vi "Configure Trigger (Edge Then Edge - Source).vi"(6 "Trigger Source Channel (0: Channel 1)":i32(ring) items=["Channel 1", "Channel 2", "Channel 3", "Channel 4", "D0", "D1", "D2", "D3", "D4", "D5", "D6", "D7", "D8", "D9", "D10", "D11", "D12", "D13", "D14", "D15"], 7 "Trigger Edge Slope (1: Positive)":i32(ring)=1 items=["Negative", "Positive"], 8 "error in (no error)":errorcluster, 9 "Arming Source Channel (0: Channel 1)":i32(ring) items=["Channel 1", "Channel 2", "Channel 3", "Channel 4", "D0", "D1", "D2", "D3", "D4", "D5", "D6", "D7", "D8", "D9", "D10", "D11", "D12", "D13", "D14", "D15"], 10 "Arming Edge Slope (1: Positive)":i32(ring)=1 items=["Negative", "Positive"], 11 "VISA resource name":refnum<visa-resource-name>) -> (0 "error out":errorcluster, 3 "VISA resource name out":refnum<visa-resource-name>)   [LabVIEW 2015, in "Agilent 2000 3000 X-Series.lvlib"]
doc: "Configures the sources of Delay(Edge Then Edge) trigger mode."
uses:
  Agilent 2000 3000 X-Series.lvlib
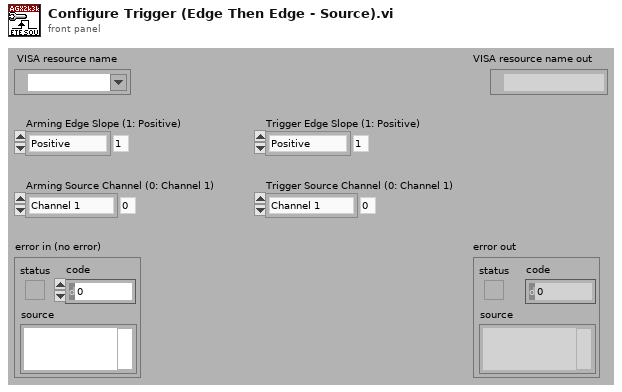
[diagram p1: front panel]
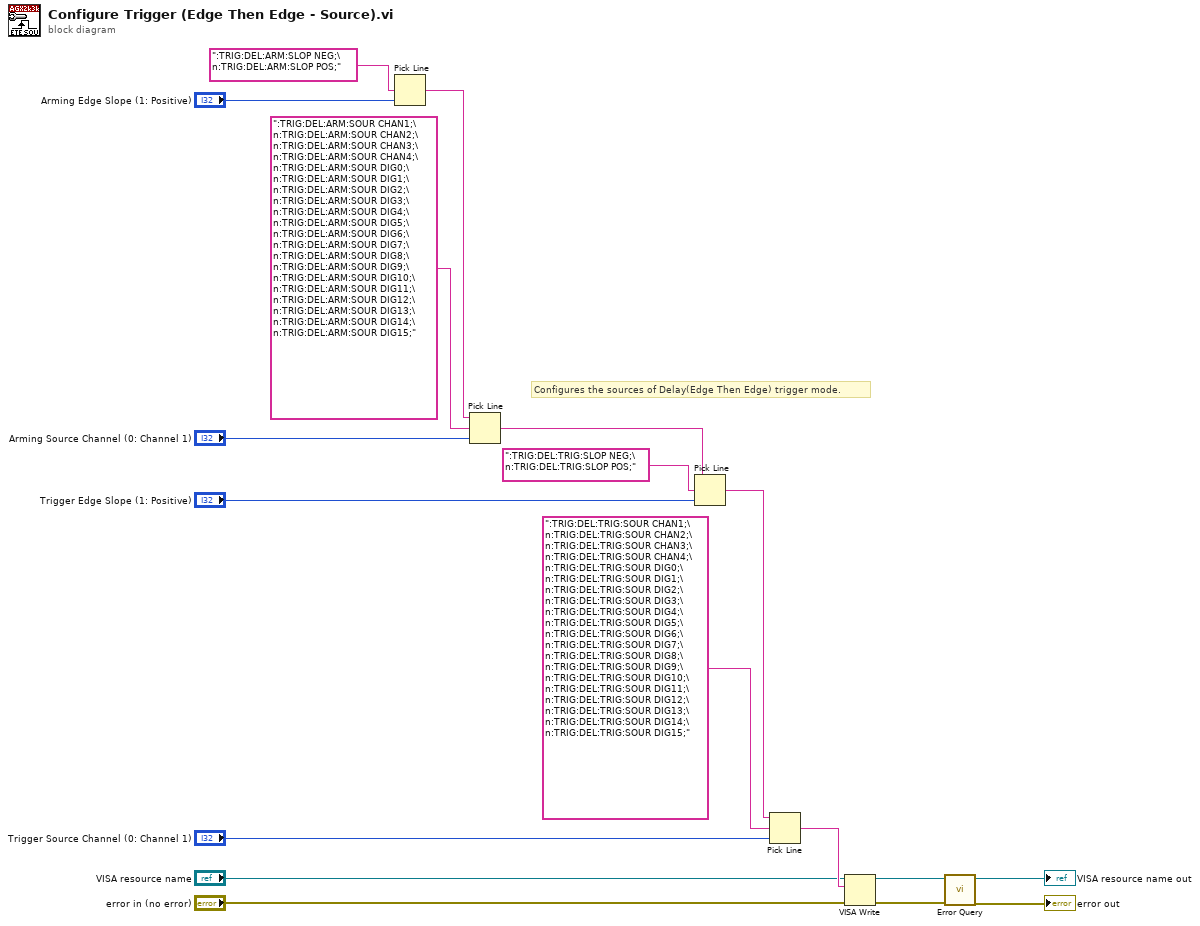
[diagram p0: block diagram]
diagram:
  # "Configures the sources of Delay(Edge Then Edge) trigger mode."
  n1 = Pick Line(multi-line string=":TRIG:DEL:ARM:SLOP NEG;\n:TRIG:DEL:ARM:SLOP POS;", line index="Arming Edge Slope (1: Positive)") -> (output string=w14:string)  [unwired: 1 out]
  n2 = Pick Line(string ("")=w14, multi-line string=":TRIG:DEL:ARM:SOUR CHAN1;\n:TRIG:DEL:ARM:SOUR CHAN2;\n:TRIG:DEL:ARM:SOUR CHAN3;\n:TRIG:DEL:ARM:SOUR CHAN4;\n:TRIG:DEL:ARM:SOUR DIG0;\n:TRIG:DEL:ARM:SOUR DIG1;\n:TRIG:DEL:ARM:SOUR DIG2;\n:TRIG:DEL:ARM:SOUR DIG3;\n:TRIG:DEL:ARM:SOUR DIG4;\n:TRIG:DEL:ARM:SOUR DIG5;\n:TRIG:DEL:ARM:SOUR DIG6;\n:TRIG:DEL:ARM:SOUR DIG7;\n:TRIG:DEL:ARM:SOUR DIG8;\n:TRIG:DEL:ARM:SOUR DIG9;\n:TRIG:DEL:ARM:SOUR DIG10;\n:TRIG:DEL:ARM:SOUR DIG11;\n:TRIG:DEL:ARM:SOUR DIG12;\n:TRIG:DEL:ARM:SOUR DIG13;\n:TRIG:DEL:ARM:SOUR DIG14;\n:TRIG:DEL:ARM:SOUR DIG15;", line index="Arming Source Channel (0: Channel 1)") -> (output string=w1:string)
  n3 = Pick Line(string ("")=w1, multi-line string=":TRIG:DEL:TRIG:SLOP NEG;\n:TRIG:DEL:TRIG:SLOP POS;", line index="Trigger Edge Slope (1: Positive)") -> (output string=w9:string)
  n4 = Pick Line(string ("")=w9, multi-line string=":TRIG:DEL:TRIG:SOUR CHAN1;\n:TRIG:DEL:TRIG:SOUR CHAN2;\n:TRIG:DEL:TRIG:SOUR CHAN3;\n:TRIG:DEL:TRIG:SOUR CHAN4;\n:TRIG:DEL:TRIG:SOUR DIG0;\n:TRIG:DEL:TRIG:SOUR DIG1;\n:TRIG:DEL:TRIG:SOUR DIG2;\n:TRIG:DEL:TRIG:SOUR DIG3;\n:TRIG:DEL:TRIG:SOUR DIG4;\n:TRIG:DEL:TRIG:SOUR DIG5;\n:TRIG:DEL:TRIG:SOUR DIG6;\n:TRIG:DEL:TRIG:SOUR DIG7;\n:TRIG:DEL:TRIG:SOUR DIG8;\n:TRIG:DEL:TRIG:SOUR DIG9;\n:TRIG:DEL:TRIG:SOUR DIG10;\n:TRIG:DEL:TRIG:SOUR DIG11;\n:TRIG:DEL:TRIG:SOUR DIG12;\n:TRIG:DEL:TRIG:SOUR DIG13;\n:TRIG:DEL:TRIG:SOUR DIG14;\n:TRIG:DEL:TRIG:SOUR DIG15;", line index="Trigger Source Channel (0: Channel 1)") -> (output string=w8:string)
  n5 = VISA Write(VISA resource name="VISA resource name", write buffer=w8, error in (no error)="error in (no error)") -> (VISA resource name out=w5:refnum<visa-resource-name>, error out=w4:errorcluster)  [unwired: 1 out]
  n6 = call "Error Query.vi"("error in (no error)"=w4, "VISA resource name"=w5) -> ("error out"=→"error out":errorcluster, "VISA resource name out"=→"VISA resource name out":refnum<visa-resource-name>)  [unwired: 8 out]
